vi "Vi ref & panel update.vi"(6 "Function":enum16{"INITIALIZE", "DEF UPDATE"}(ring)=enum."DEF UPDATE", 8 "error in (no error)":errorcluster, 10 "Defer Panel Updates":bool, 11 "VI ref in":refnum<vi>) -> (0 "error out":errorcluster, 3 "VI ref out":refnum<vi>)   [LabVIEW 2019]
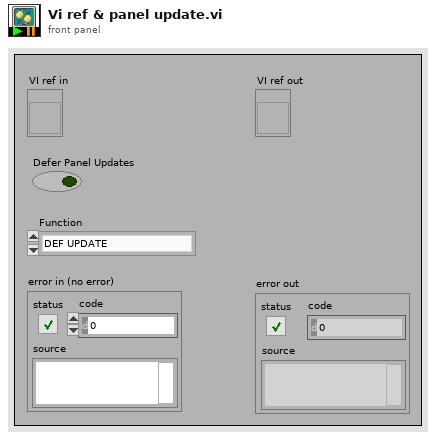
[diagram p1: front panel]
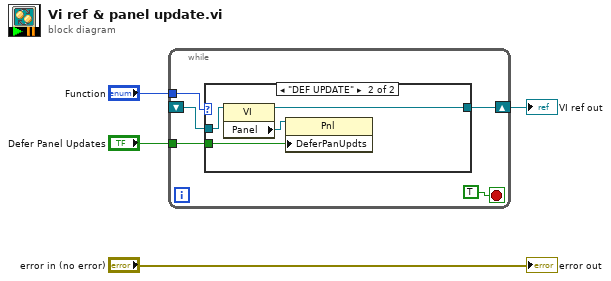
[diagram p0: block diagram]
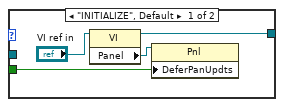
[diagram p2: hidden frame]
diagram:
  n1 = while {
    tunnel: "Defer Panel Updates" -> [w9]
    tunnel: "Function" -> [w6]
    shift-right: [w5] -> w2
    shift-left: _ -> [w8]
    stop <- TRUE stop-if-true
    n2 = case shown="\"DEF UPDATE\"" w6 {
      tunnel: w9 -> [w11 w14]
      tunnel: w8 -> [_ w16]
      tunnel: [w10 w15] -> w5
      frame "INITIALIZE", Default {
        n3 = property class="VI"(reference="VI ref in") -> (reference out=w10:refnum<vi>, "Panel"=w13:refnum<vi>)  [unwired: 1 in, 1 out]
        n4 = property class="Pnl"(reference=w13, "DeferPanUpdts"=w11) -> ()  [unwired: 1 in, 2 out]
      }
      frame "DEF UPDATE" {
        n5 = property class="VI"(reference=w16) -> (reference out=w15:refnum<vi>, "Panel"=w17:refnum<vi>)  [unwired: 1 in, 1 out]
        n6 = property class="Pnl"(reference=w17, "DeferPanUpdts"=w14) -> ()  [unwired: 1 in, 2 out]
      }
    }
  }
  "VI ref out" <- w2
  "error out" <- "error in (no error)"
